vi "get_frame_properties.vi"(8 "error in (no error)":errorcluster, 11 "ScanModeTS090821Circular2D in":refnum<class "ImagingModeTS090821Circular2D.lvclass">) -> (0 "error out":errorcluster, 1 "pixels per line":i32, 2 "lines per frame":i32, 3 "ScanModeTS090821Circular2D out":refnum<class "ImagingModeTS090821Circular2D.lvclass">, 4 "number of frames":i32)   [LabVIEW 2010, in "ImagingModeTS090821Circular2D.lvclass"]
uses:
  ImagingModeTS090821Circular2D.lvclass
  ImagingModeTS090821Circular2D.lvclass/ImagingModeTS090821Circular2D.ctl
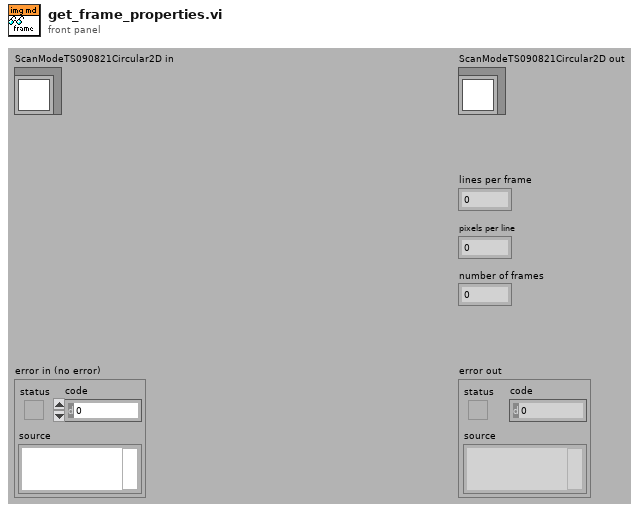
[diagram p1: front panel]
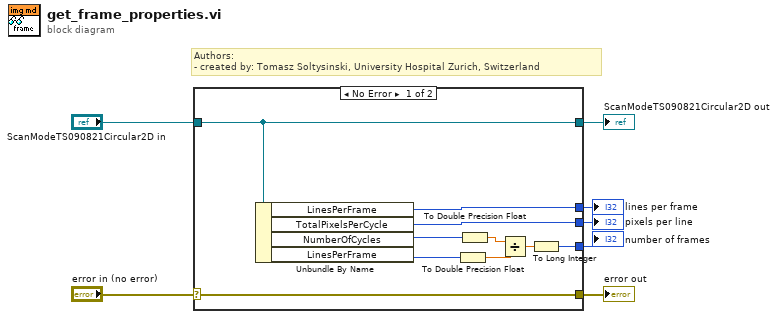
[diagram p0: block diagram]
diagram:
  # "Authors: \n- created by: Tomasz Soltysinski, University Hospital Zurich, Switzerland"
  n1 = case shown="No Error" "error in (no error)" {
    selector: "error in (no error)" -> [w17 w18]
    tunnel: [w17 w18] -> w6
    tunnel: [w16 w19] -> w4
    tunnel: "ScanModeTS090821Circular2D in" -> [w16 w19]
    tunnel: [w15 _] -> w3
    tunnel: [w14 _] -> w2
    tunnel: [w8 _] -> w1
    frame No Error {
      n2 = Unbundle By Name(w16) -> ("LinesPerFrame"=w15:i32, "TotalPixelsPerCycle"=w14:i32, "NumberOfCycles"=w13:i32, "LinesPerFrame"=w12:i32)
      n3 = To Double Precision Float(number=w12) -> (double precision float=w11:dbl)
      n4 = To Double Precision Float(number=w13) -> (double precision float=w10:dbl)
      n5 = Divide(x=w10, y=w11) -> (x/y=w9:dbl)
      n6 = To Long Integer(number=w9) -> (32bit integer=w8:i32)
    }
    frame Error {
    }
  }
  "error out" <- w6
  "ScanModeTS090821Circular2D out" <- w4
  "lines per frame" <- w3
  "pixels per line" <- w2
  "number of frames" <- w1
